vi "T7 TCP Open KAG.vi"(8 "error in":errorcluster, 11 "IP Configuration":T1={"Device IP"="192.168.126.147", "Port"=502}) -> (0 "error out":errorcluster, 3 "connection ID out":refnum<k5>)   [LabVIEW 2022 SP3]
doc: "TCP Open to read data from socket 702"
uses:
  T7 IP Config KAG.ctl
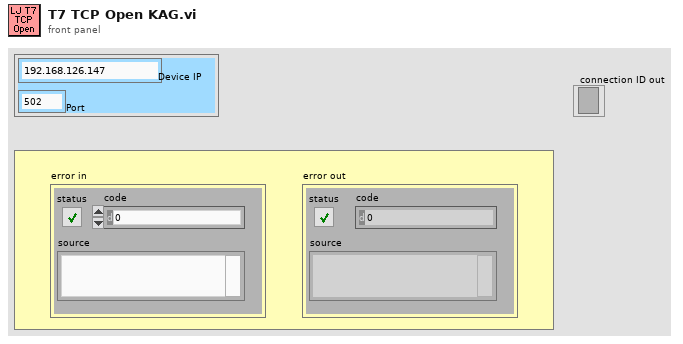
[diagram p1: front panel]
types:
  T1 = typedef "T7 IP Config KAG.ctl" = cluster{"Device IP":string, "Port":i32}
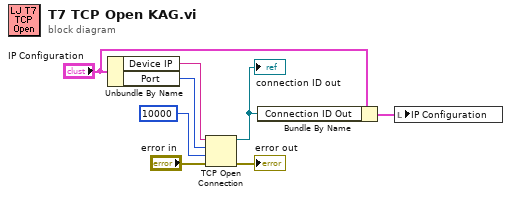
[diagram p0: block diagram]
diagram:
  n1 = Unbundle By Name("IP Configuration") -> ("Device IP"=w7:string, "Port"=w6:i32)
  n2 = TCP Open Connection(address=w7, remote port or service name=w6, timeout ms (60000)=10000, error in (no error)="error in") -> (connection ID=w1:refnum<k5>, error out=→"error out":errorcluster)  [unwired: 1 out]
  "connection ID out" <- w1
  n3 = Bundle By Name(cluster="IP Configuration", "Connection ID Out"=w1) -> (w2:T1)
  n4 = local write "IP Configuration"(w2) -> ()
